vi "quiz1.vi"() -> ()   [LabVIEW 2020]
uses:
  <vilib>/Utility/error.llb/whitespace.ctl
panel:
  in  "Array 3":string[](array[string])
  in  "Array 2":string[](array[string])
  in  "Array":string[](array[string])
  in  "Numeric 2":i64
  out "led 3":bool
  in  "swiche 3":bool
  out "led 2":bool
  in  "swiche 2":bool
  in  "swiche 1":bool
  out "led1":bool
  out "Numeric":i64
  out "number":dbl
  out "Salida de comandos":string
  in  "Ingreso de trama":string
  in  "Ingreso de comandos":string
  in  "Button":bool
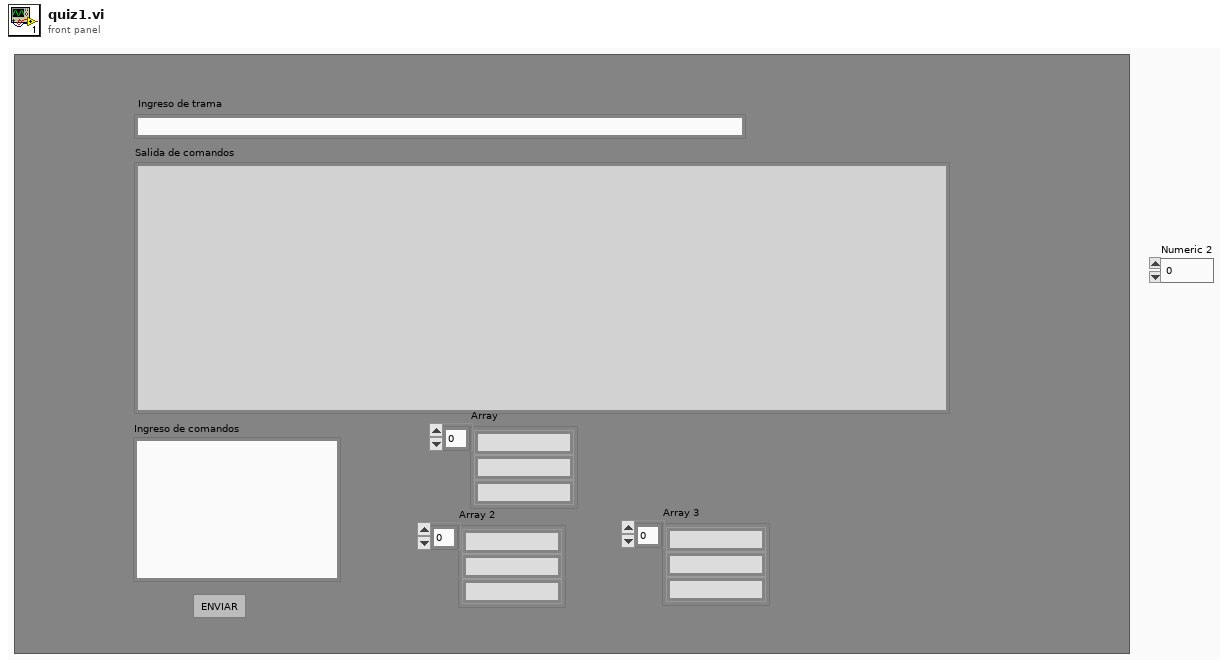
[diagram p1: front panel]
types:
  T1 = enum8{"Enabled", "Disabled", "Disabled and Grayed Out"}
  T2 = typedef "whitespace.ctl" = u16
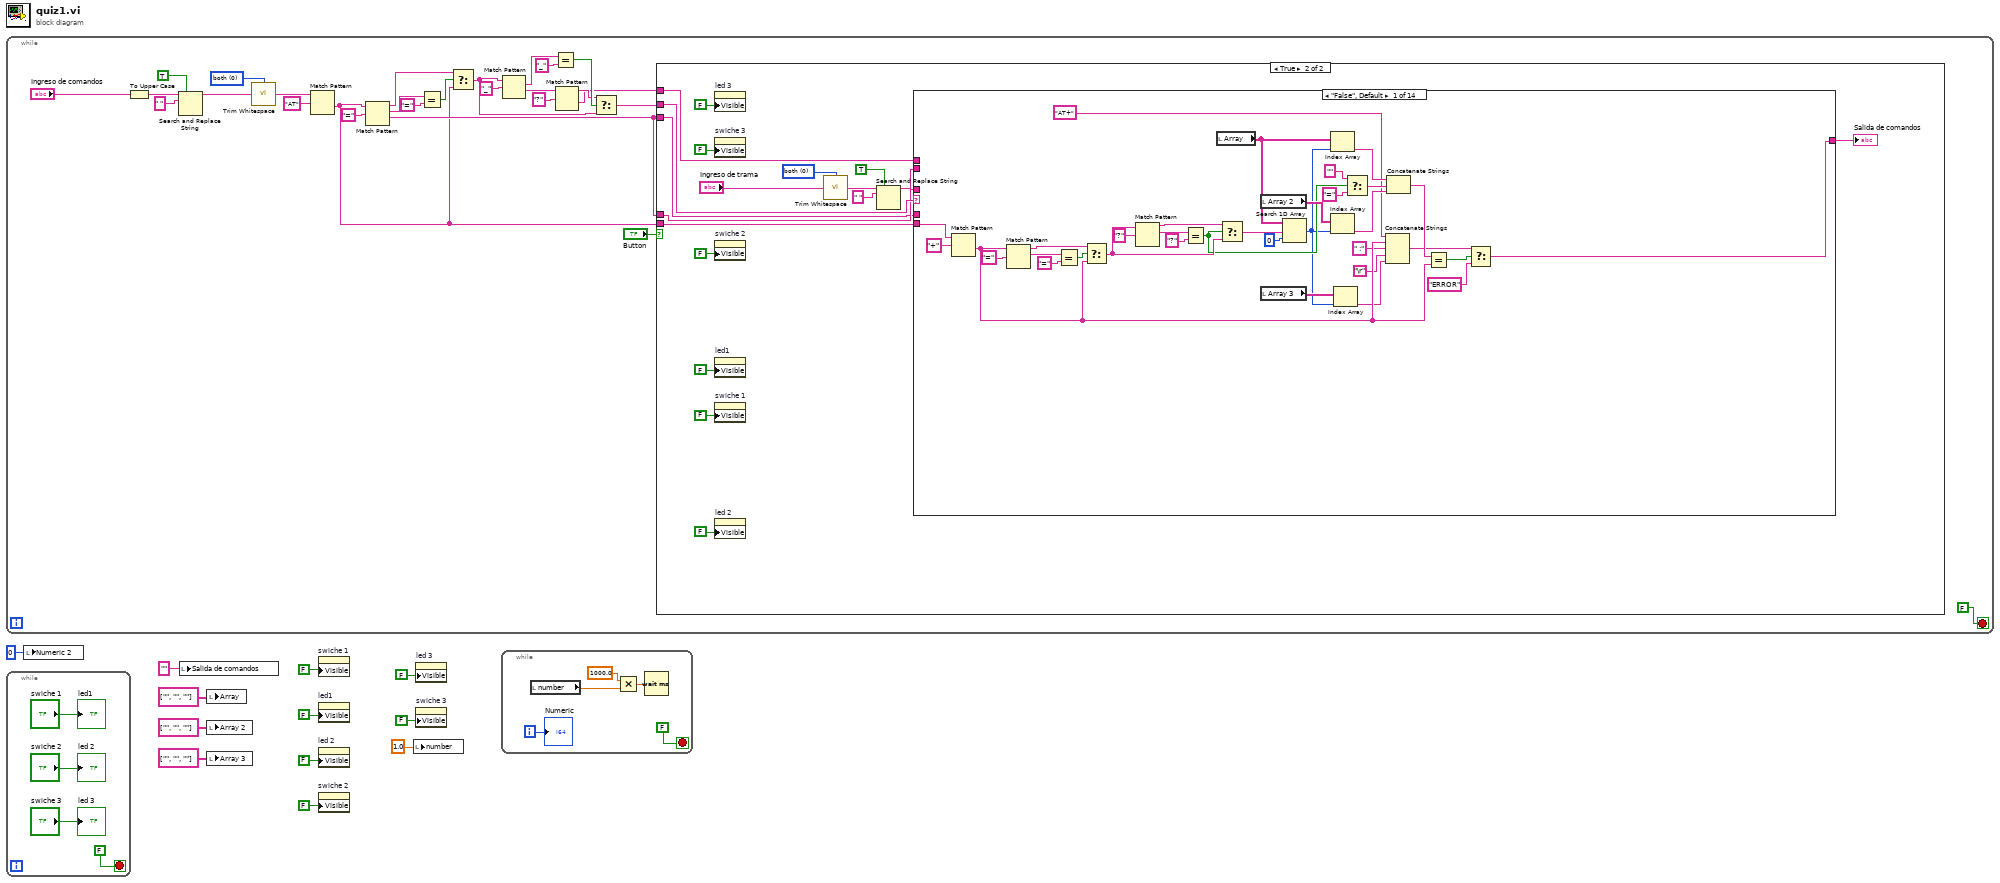
[diagram p0: block diagram]
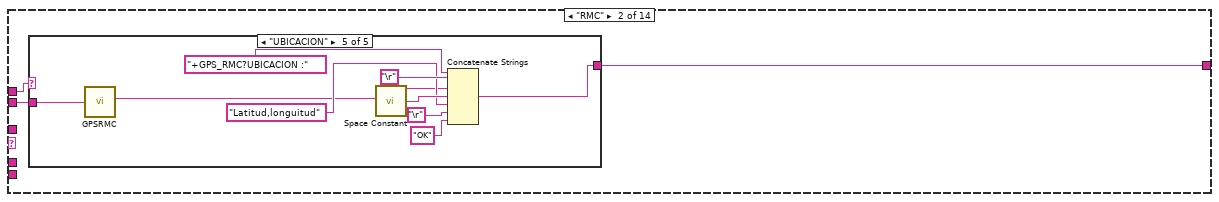
[diagram p3: hidden frame]
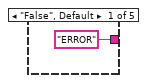
[diagram p4: hidden frame]
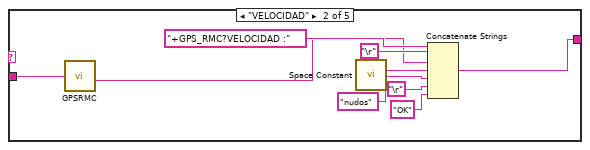
[diagram p5: hidden frame]
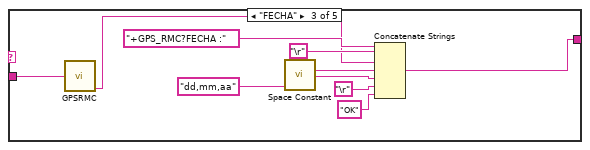
[diagram p6: hidden frame]
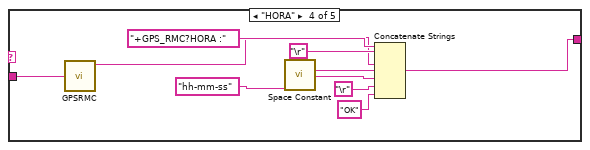
[diagram p7: hidden frame]
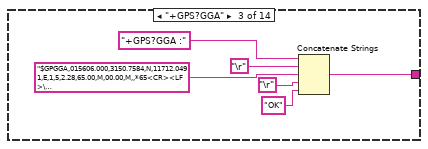
[diagram p8: hidden frame]
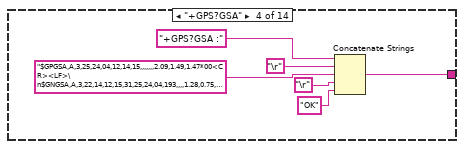
[diagram p9: hidden frame]
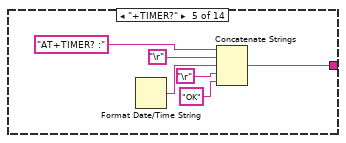
[diagram p10: hidden frame]
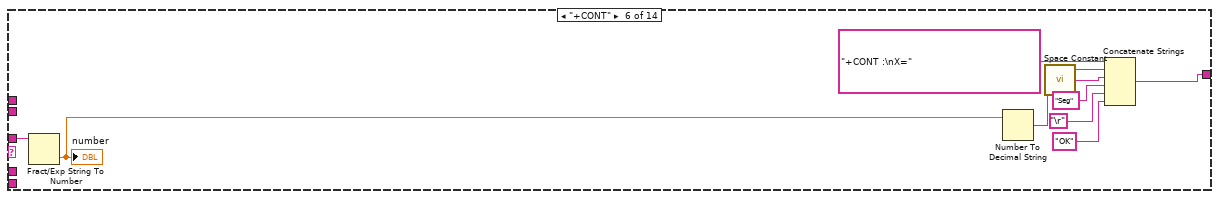
[diagram p11: hidden frame]
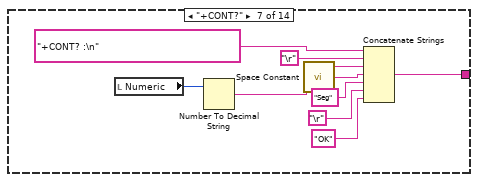
[diagram p12: hidden frame]
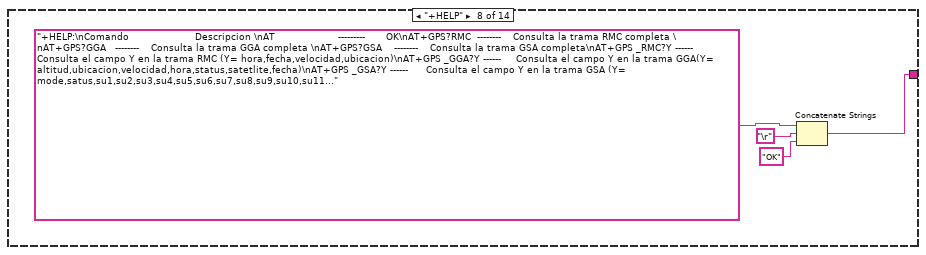
[diagram p13: hidden frame]
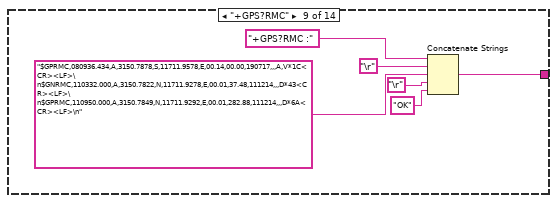
[diagram p14: hidden frame]
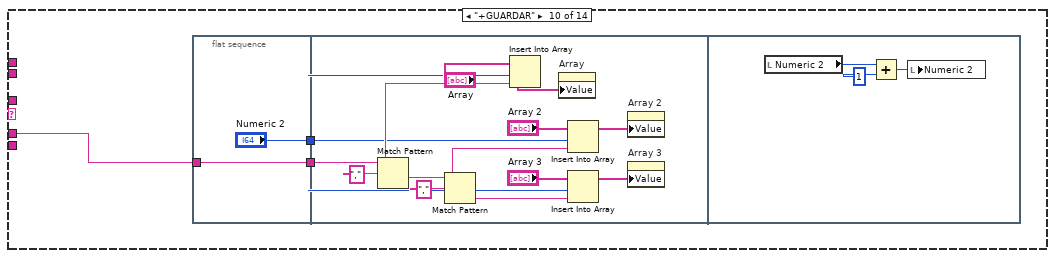
[diagram p15: hidden frame]
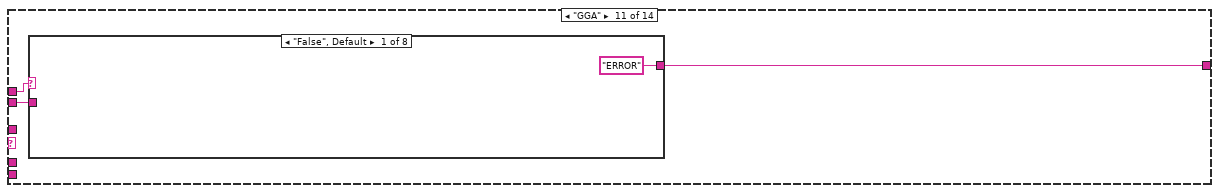
[diagram p16: hidden frame]
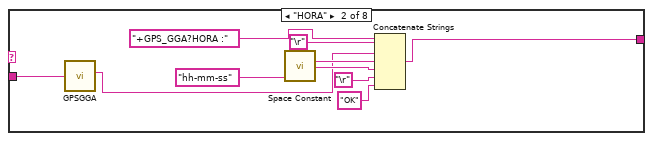
[diagram p17: hidden frame]
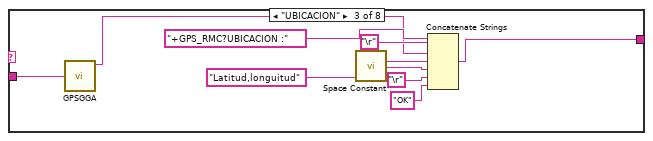
[diagram p18: hidden frame]
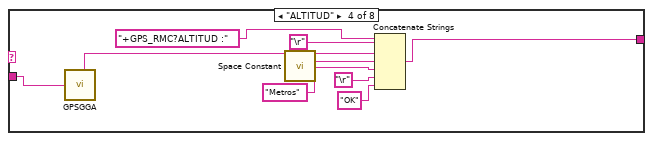
[diagram p19: hidden frame]
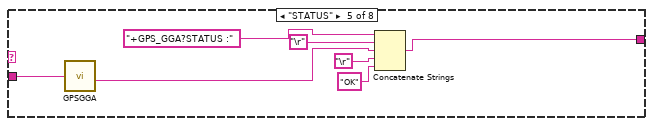
[diagram p20: hidden frame]
diagram:
  n1 = while {
    stop <- FALSE stop-if-true
    w19 = T2 0 items=["both", "start of string", "end of string"] ("location (both)")
    n2 = To Upper Case(1:"Ingreso de comandos") -> (0:w23:string)
    n3 = Search and Replace String(replace all?=TRUE ("replace all? (F)"), input string=w23, search string=" ") -> (result string=w21:string)  [unwired: 5 in, 3 out]
    n4 = call <vilib>:"Trim Whitespace.vi"("string"=w21, "location (both)"=w19) -> ("trimmed string"=w17:string)
    n5 = Match Pattern(string=w17, regular expression="AT") -> (after substring=w13:string)  [unwired: 1 in, 3 out]
    n6 = Match Pattern(string=w13, regular expression="=") -> (before substring=w33:string, match substring=w35:string, after substring=w14:string)  [unwired: 1 in, 1 out]
    n7 = Equal?(x=w35, y="=") -> (x = y?=w32:bool)
    n8 = Select(t=w33, s=w32, f=w13) -> (s? t:f=w27:string)
    n9 = Match Pattern(string=w27, regular expression="_") -> (match substring=w30:string, after substring=w26:string)  [unwired: 1 in, 2 out]
    n10 = Equal?(x=w30, y="_") -> (x = y?=w28:bool)
    n11 = Match Pattern(string=w26, regular expression="?") -> (before substring=w24:string, after substring=w16:string)  [unwired: 1 in, 2 out]
    n12 = Select(t=w24, s=w28, f=w27) -> (s? t:f=w15:string)
    n13 = case shown="True" "Button" {
      tunnel: w14 -> [_ w55]
      tunnel: w15 -> [_ w56]
      tunnel: w16 -> [_ w54]
      tunnel: w14 -> [_ w41]
      tunnel: w13 -> [_ w40]
      frame False {
      }
      frame True {
        w48 = T2 0 items=["both", "start of string", "end of string"] ("location (both)")
        n14 = property on="led 3" class="Bool (strict)"("Visible"=FALSE) -> ()  [unwired: 2 in, 2 out]
        n15 = property on="swiche 3" class="Bool (strict)"("Visible"=FALSE) -> ()  [unwired: 2 in, 2 out]
        n16 = property on="swiche 2" class="Bool (strict)"("Visible"=FALSE) -> ()  [unwired: 2 in, 2 out]
        n17 = property on="led1" class="Bool (strict)"("Visible"=FALSE) -> ()  [unwired: 2 in, 2 out]
        n18 = property on="swiche 1" class="Bool (strict)"("Visible"=FALSE) -> ()  [unwired: 2 in, 2 out]
        n19 = property on="led 2" class="Bool (strict)"("Visible"=FALSE) -> ()  [unwired: 2 in, 2 out]
        n20 = call <vilib>:"Trim Whitespace.vi"("string"="Ingreso de trama", "location (both)"=w48) -> ("trimmed string"=w50:string)
        n21 = Search and Replace String(replace all?=TRUE ("replace all? (F)"), input string=w50, search string=" ") -> (result string=w49:string)  [unwired: 5 in, 3 out]
        n22 = case shown="\"False\", Default" w56 {
          tunnel: [w63 w92 w132 w138 w149 w154 w163 w168 w172 _ w201 w262 w390 w403] -> w57
          tunnel: w49 -> [_ w93 _ _ _ _ _ _ _ _ w200 w260 _ _]
          tunnel: w55 -> [_ _ _ _ _ w158 _ _ _ _ _ _ _ _]
          tunnel: w54 -> [_ w94 _ _ _ _ _ _ _ _ w202 w261 _ _]
          tunnel: w41 -> [_ _ _ _ _ _ _ _ _ w179 _ _ _ _]
          tunnel: w40 -> [w91 _ _ _ _ _ _ _ _ _ _ _ _ _]
          frame "False", Default {
            n23 = Match Pattern(string=w91, regular expression="+") -> (after substring=w65:string)  [unwired: 1 in, 3 out]
            n24 = Match Pattern(string=w65, regular expression="=") -> (before substring=w85:string, match substring=w88:string)  [unwired: 1 in, 2 out]
            n25 = Equal?(x=w88, y="=") -> (x = y?=w86:bool)
            n26 = Select(t=w85, s=w86, f=w65) -> (s? t:f=w78:string)
            n27 = Match Pattern(string=w78, regular expression="?") -> (before substring=w81:string, match substring=w83:string)  [unwired: 1 in, 2 out]
            n28 = Equal?(x=w83, y="?") -> (x = y?=w74:bool)
            n29 = local read "Array"() -> (w77:string[])
            n30 = Select(t=w81, s=w74, f=w78) -> (s? t:f=w80:string)
            n31 = local read "Array 2"() -> (w76:string[])
            n32 = local read "Array 3"() -> (w69:string[])
            n33 = Search 1D Array(1D array=w77, element=w80, start index (0)=0) -> (index of element=w58:i32)
            n34 = Index Array(array=w77, index=w58) -> (element=w75:string)
            n35 = Index Array(array=w76, index=w58) -> (element=w70:string)
            n36 = Index Array(array=w69, index=w58) -> (element=w62:string)
            n37 = Select(t="", s=w74, f="=") -> (s? t:f=w71:string)
            n38 = Concatenate Strings("AT+" ("string"), w65, " :" ("string"), "\r", w62) -> (w64:string)
            n39 = Concatenate Strings(w75, w71, w70) -> (w68:string)
            n40 = Equal?(x=w68, y=w65) -> (x = y?=w67:bool)
            n41 = Select(t=w64, s=w67, f="ERROR") -> (s? t:f=w63:string)
          }
          frame "RMC" {
            n42 = case shown="\"UBICACION\"" w94 {
              tunnel: w93 -> [_ w104 w113 w122 w131]
              tunnel: ["ERROR" w96 w109 w114 w124] -> w92
              frame "False", Default {
              }
              frame "VELOCIDAD" {
                n43 = call "GPSRMC.vi"("String"=w104) -> ("Velocidad"=w100:string)  [unwired: 3 out]
                n44 = call <vilib>:"Space Constant.vi"() -> ("String"=w103:string)
                n45 = Concatenate Strings("+GPS_RMC?VELOCIDAD :", "\r", w100, w103, "nudos" ("string"), "\r", "OK" ("string")) -> (w96:string)
              }
              frame "FECHA" {
                n46 = call "GPSRMC.vi"("String"=w113) -> ("Fecha"=w110:string)  [unwired: 3 out]
                n47 = call <vilib>:"Space Constant.vi"() -> ("String"=w108:string)
                n48 = Concatenate Strings("+GPS_RMC?FECHA :", "\r", w110, w108, "dd,mm,aa" ("string"), "\r", "OK" ("string")) -> (w109:string)
              }
              frame "HORA" {
                n49 = call "GPSRMC.vi"("String"=w122) -> ("Hora"=w115:string)  [unwired: 3 out]
                n50 = call <vilib>:"Space Constant.vi"() -> ("String"=w121:string)
                n51 = Concatenate Strings("+GPS_RMC?HORA :", "\r", w115, w121, "hh-mm-ss" ("string"), "\r", "OK" ("string")) -> (w114:string)
              }
              frame "UBICACION" {
                n52 = call "GPSRMC.vi"("String"=w131) -> ("Ubicación"=w123:string)  [unwired: 3 out]
                n53 = call <vilib>:"Space Constant.vi"() -> ("String"=w130:string)
                n54 = Concatenate Strings("+GPS_RMC?UBICACION :", "\r", w123, w130, "Latitud,longuitud" ("string"), "\r", "OK" ("string")) -> (w124:string)
              }
            }
          }
          frame "+GPS?GGA" {
            n55 = Concatenate Strings("+GPS?GGA :" ("string"), "\r", "$GPGGA,015606.000,3150.7584,N,11712.0491,E,1,5,2.28,65.00,M,00.00,M,,*65<CR><LF>\n$GNGGA,083354.000,3150.7790,N,11711.9289,E,1,8,2.85,53.20,M,00.00,M,,*4B<CR><LF>", "\r", "OK" ("string")) -> (w132:string)
          }
          frame "+GPS?GSA" {
            n56 = Concatenate Strings("+GPS?GSA :" ("string"), "\r", "$GPGSA,A,3,25,24,04,12,14,15,,,,,,,2.09,1.49,1.47*00<CR><LF>\n$GNGSA,A,3,22,14,12,15,31,25,24,04,193,,,,1.28,0.75,1.03*29<CR><LF>\n$GPGSA,A,3,03,17,09,23,,,,,,,,,3.65,3.51,0.99,1*15<CR><LF>\n$GNGSA,A,3,09,17,19,06,23,,,,,,,,2.20,1.97,0.98,1*0F<CR><LF>", "\r", "OK" ("string")) -> (w138:string)
          }
          frame "+TIMER?" {
            n57 = Format Date/Time String() -> (date/time string=w146:string)  [unwired: 3 in]
            n58 = Concatenate Strings("AT+TIMER? :", "\r", w146, "\r", "OK" ("string")) -> (w149:string)
          }
          frame "+CONT" {
            n59 = Fract/Exp String To Number(string=w158) -> (number=w156:dbl)  [unwired: 3 in, 1 out]
            "number" <- w156
            n60 = Number To Decimal String(number=w156) -> (decimal integer string=w155:string)  [unwired: 1 in]
            n61 = call <vilib>:"Space Constant.vi"() -> ("String"=w153:string)
            n62 = Concatenate Strings("+CONT :\nX=", w155, w153, "Seg" ("string"), "\r", "OK" ("string")) -> (w154:string)
          }
          frame "+CONT?" {
            n63 = local read "Numeric"() -> (w167:i64)
            n64 = Number To Decimal String(number=w167) -> (decimal integer string=w164:string)  [unwired: 1 in]
            n65 = call <vilib>:"Space Constant.vi"() -> ("String"=w159:string)
            n66 = Concatenate Strings("+CONT? :\n", "\r", w164, w159, "Seg" ("string"), "\r", "OK" ("string")) -> (w163:string)
          }
          frame "+HELP" {
            n67 = Concatenate Strings("+HELP:\nComando                      Descripcion \nAT                     ---------       OK\nAT+GPS?RMC  --------    Consulta la trama RMC completa \nAT+GPS?GGA   --------    Consulta la trama GGA completa \nAT+GPS?GSA    --------    Consulta la trama GSA completa\nAT+GPS _RMC?Y ------    Consulta el campo Y en la trama RMC (Y= hora,fecha,velocidad,ubicacion)\nAT+GPS _GGA?Y ------     Consulta el campo Y en la trama GGA(Y= altitud,ubicacion,velocidad,hora,status,satetlite,fecha)\nAT+GPS _GSA?Y ------      Consulta el campo Y en la trama GSA (Y= mode,satus,su1,su2,su3,su4,su5,su6,su7,su8,su9,su10,su11,su12)\nAT+TIMER?           --------  Consulta la hora y fecha del sistema\nAT+CONT=X      --------- Modifica el tiempo de incremento del contador en X tiempo \nAT+CONT?         ----------Lee  la variable del contador \nAT+ESTADO?     ----------Lee el estado de los leds y pulsadores\nAT+CAMBIAR   ---------  Modifica el estado de los leds y el pulsador", "\r", "OK" ("string")) -> (w168:string)
          }
          frame "+GPS?RMC" {
            n68 = Concatenate Strings("+GPS?RMC :" ("string"), "\r", "$GPRMC,080936.434,A,3150.7878,S,11711.9578,E,00.14,00.00,190717,,,A,V*1C<CR><LF>\n$GNRMC,110332.000,A,3150.7822,N,11711.9278,E,00.01,37.48,111214,,,D*43<CR><LF>\n$GPRMC,110950.000,A,3150.7849,N,11711.9292,E,00.01,282.88,111214,,,D*6A<CR><LF>\n", "\r", "OK" ("string")) -> (w172:string)
          }
          frame "+GUARDAR" {
            n69 = flat-sequence {
              tunnel: ["Numeric 2"] -> w180
              tunnel: w179 -> [w181]
              tunnel: [w181] -> w178
              tunnel: w180 -> [w184]
              tunnel: w178 -> [w196]
              frame #0 {
              }
              frame #1 {
                n70 = Match Pattern(string=w196, regular expression=",") -> (before substring=w194:string, after substring=w189:string)  [unwired: 1 in, 2 out]
                n71 = Match Pattern(string=w189, regular expression=",") -> (before substring=w187:string, after substring=w185:string)  [unwired: 1 in, 2 out]
                n72 = Insert Into Array(array="Array", index=w184, new element=w194) -> (w191:string[])
                n73 = property on="Array" class="Arr (strict)"("Value"=w191) -> ()  [unwired: 2 in, 2 out]
                n74 = Insert Into Array(array="Array 2", index=w184, new element=w187) -> (w190:string[])
                n75 = Insert Into Array(array="Array 3", index=w184, new element=w185) -> (w183:string[])
                n76 = property on="Array 2" class="Arr (strict)"("Value"=w190) -> ()  [unwired: 2 in, 2 out]
                n77 = property on="Array 3" class="Arr (strict)"("Value"=w183) -> ()  [unwired: 2 in, 2 out]
              }
              frame #2 {
                n78 = local read "Numeric 2"() -> (w199:i64)
                n79 = Add(x=w199, y=i64 1) -> (x+y=w197:i64)
                n80 = local write "Numeric 2"(w197) -> ()
              }
            }
          }
          frame "GGA" {
            n81 = case shown="\"False\", Default" w202 {
              tunnel: ["ERROR" w206 w214 w222 w233 w238 w248 w254] -> w201
              tunnel: w200 -> [_ w204 w213 w223 w237 w246 w253 _]
              frame "False", Default {
              }
              frame "HORA" {
                n82 = call "GPSGGA.vi"("String"=w204) -> ("Hora"=w205:string)  [unwired: 5 out]
                n83 = call <vilib>:"Space Constant.vi"() -> ("String"=w212:string)
                n84 = Concatenate Strings("+GPS_GGA?HORA :", "\r", w205, w212, "hh-mm-ss" ("string"), "\r", "OK" ("string")) -> (w206:string)
              }
              frame "UBICACION" {
                n85 = call "GPSGGA.vi"("String"=w213) -> ("Ubicación"=w215:string)  [unwired: 5 out]
                n86 = call <vilib>:"Space Constant.vi"() -> ("String"=w221:string)
                n87 = Concatenate Strings("+GPS_RMC?UBICACION :", "\r", w215, w221, "Latitud,longuitud" ("string"), "\r", "OK" ("string")) -> (w214:string)
              }
              frame "ALTITUD" {
                n88 = call "GPSGGA.vi"("String"=w223) -> ("Altitud"=w224:string)  [unwired: 5 out]
                n89 = call <vilib>:"Space Constant.vi"() -> ("String"=w230:string)
                n90 = Concatenate Strings("+GPS_RMC?ALTITUD :", "\r", w224, w230, "Metros" ("string"), "\r", "OK" ("string")) -> (w222:string)
              }
              frame "STATUS" {
                n91 = call "GPSGGA.vi"("String"=w237) -> ("Fix Status"=w236:string)  [unwired: 5 out]
                n92 = Concatenate Strings("+GPS_GGA?STATUS :" ("string"), "\r", w236, "\r", "OK" ("string")) -> (w233:string)
              }
              frame "GEOIDE" {
                n93 = call "GPSGGA.vi"("String"=w246) -> ("Sep Geoide"=w239:string)  [unwired: 5 out]
                n94 = call <vilib>:"Space Constant.vi"() -> ("String"=w245:string)
                n95 = Concatenate Strings("+GPS_RMC?GEOIDE :", "\r", w239, w245, "Metros" ("string"), "\r", "OK" ("string")) -> (w238:string)
              }
              frame "SATELITE" {
                n96 = call "GPSGGA.vi"("String"=w253) -> ("# Satelite"=w249:string)  [unwired: 5 out]
                n97 = Concatenate Strings("+GPS_GGA?SATELITE :" ("string"), "\r", w249, "\r", "OK" ("string")) -> (w248:string)
              }
              frame "VELOCIDAD" {
                n98 = Concatenate Strings("+GPS_GGA?VELOCIDAD :" ("string"), "\r", "La trama GGA no tiene velocidad", "\r", "OK" ("string")) -> (w254:string)
              }
            }
          }
          frame "GSA" {
            n99 = case shown="\"False\", Default" w261 {
              tunnel: ["ERROR -CAMPO NO ENCONTRADO" w265 w274 w282 w291 w300 w310 w319 w328 w336 w345 w355 w363 w372 w382] -> w262
              tunnel: w260 -> [_ w264 w273 w283 w292 w301 w309 w318 w327 w337 w346 w354 w364 w373 w381]
              frame "False", Default {
              }
              frame "MODO" {
                n100 = call "GPSGSA.vi"("string"=w264) -> ("Array"=w272:string[])
                n101 = Index Array(array=w272, index=0) -> (element=w266:string)
                n102 = Concatenate Strings("+GPS_GSA?MODO :" ("string"), "\r", w266, "\r", "OK" ("string")) -> (w265:string)
              }
              frame "STATUS" {
                n103 = call "GPSGSA.vi"("string"=w273) -> ("Array"=w281:string[])
                n104 = Index Array(array=w281, index=1) -> (element=w275:string)
                n105 = Concatenate Strings("+GPS_GSA?STATUS :" ("string"), "\r", w275, "\r", "OK" ("string")) -> (w274:string)
              }
              frame "SATELITE1" {
                n106 = call "GPSGSA.vi"("string"=w283) -> ("Array"=w290:string[])
                n107 = Index Array(array=w290, index=2) -> (element=w284:string)
                n108 = Concatenate Strings("+GPS_GSA?SATELITE1 :" ("string"), "\r", w284, "\r", "OK" ("string")) -> (w282:string)
              }
              frame "SATELITE2" {
                n109 = call "GPSGSA.vi"("string"=w292) -> ("Array"=w299:string[])
                n110 = Index Array(array=w299, index=3) -> (element=w293:string)
                n111 = Concatenate Strings("+GPS_GSA?SATELITE2 :" ("string"), "\r", w293, "\r", "OK" ("string")) -> (w291:string)
              }
              frame "SATELITE3" {
                n112 = call "GPSGSA.vi"("string"=w301) -> ("Array"=w308:string[])
                n113 = Index Array(array=w308, index=4) -> (element=w302:string)
                n114 = Concatenate Strings("+GPS_GSA?SATELITE3 :" ("string"), "\r", w302, "\r", "OK" ("string")) -> (w300:string)
              }
              frame "SATELITE4" {
                n115 = call "GPSGSA.vi"("string"=w309) -> ("Array"=w317:string[])
                n116 = Index Array(array=w317, index=5) -> (element=w311:string)
                n117 = Concatenate Strings("+GPS_GSA?SATELITE4 :" ("string"), "\r", w311, "\r", "OK" ("string")) -> (w310:string)
              }
              frame "SATELITE5" {
                n118 = call "GPSGSA.vi"("string"=w318) -> ("Array"=w326:string[])
                n119 = Index Array(array=w326, index=6) -> (element=w320:string)
                n120 = Concatenate Strings("+GPS_GSA?SATELITE5 :" ("string"), "\r", w320, "\r", "OK" ("string")) -> (w319:string)
              }
              frame "SATELITE9" {
                n121 = call "GPSGSA.vi"("string"=w327) -> ("Array"=w335:string[])
                n122 = Index Array(array=w335, index=10) -> (element=w329:string)
                n123 = Concatenate Strings("+GPS_GSA?SATELITE9 :" ("string"), "\r", w329, "\r", "OK" ("string")) -> (w328:string)
              }
              frame "SATELITE11" {
                n124 = call "GPSGSA.vi"("string"=w337) -> ("Array"=w344:string[])
                n125 = Index Array(array=w344, index=12) -> (element=w338:string)
                n126 = Concatenate Strings("+GPS_GSA?SATELITE11 :" ("string"), "\r", w338, "\r", "OK" ("string")) -> (w336:string)
              }
              frame "SATELITE10" {
                n127 = call "GPSGSA.vi"("string"=w346) -> ("Array"=w353:string[])
                n128 = Index Array(array=w353, index=11) -> (element=w347:string)
                n129 = Concatenate Strings("+GPS_GSA?SATELITE10 :" ("string"), "\r", w347, "\r", "OK" ("string")) -> (w345:string)
              }
              frame "SATELITE12" {
                n130 = call "GPSGSA.vi"("string"=w354) -> ("Array"=w362:string[])
                n131 = Index Array(array=w362, index=13) -> (element=w356:string)
                n132 = Concatenate Strings("+GPS_GSA?SATELITE12 :" ("string"), "\r", w356, "\r", "OK" ("string")) -> (w355:string)
              }
              frame "SATELITE7" {
                n133 = call "GPSGSA.vi"("string"=w364) -> ("Array"=w371:string[])
                n134 = Index Array(array=w371, index=8) -> (element=w365:string)
                n135 = Concatenate Strings("+GPS_GSA?SATELITE7 :" ("string"), "\r", w365, "\r", "OK" ("string")) -> (w363:string)
              }
              frame "SATELITE6" {
                n136 = call "GPSGSA.vi"("string"=w373) -> ("Array"=w380:string[])
                n137 = Index Array(array=w380, index=7) -> (element=w374:string)
                n138 = Concatenate Strings("+GPS_GSA?SATELITE6 :" ("string"), "\r", w374, "\r", "OK" ("string")) -> (w372:string)
              }
              frame "SATELITE8" {
                n139 = call "GPSGSA.vi"("string"=w381) -> ("Array"=w389:string[])
                n140 = Index Array(array=w389, index=9) -> (element=w383:string)
                n141 = Concatenate Strings("+GPS_GSA?SATELITE8 :" ("string"), "\r", w383, "\r", "OK" ("string")) -> (w382:string)
              }
            }
          }
          frame "+ESTADO?" {
            n142 = property on="swiche 1" class="Bool (strict)"("Visible"=TRUE) -> ()  [unwired: 2 in, 2 out]
            n143 = property on="swiche 2" class="Bool (strict)"("Visible"=TRUE) -> ()  [unwired: 2 in, 2 out]
            n144 = property on="swiche 3" class="Bool (strict)"("Visible"=TRUE) -> ()  [unwired: 2 in, 2 out]
            n145 = property on="led 3" class="Bool (strict)"("Visible"=TRUE) -> ()  [unwired: 2 in, 2 out]
            n146 = property on="led 2" class="Bool (strict)"("Visible"=TRUE) -> ()  [unwired: 2 in, 2 out]
            n147 = property on="led1" class="Bool (strict)"("Visible"=TRUE) -> ()  [unwired: 2 in, 2 out]
            n148 = property on="swiche 3" class="Bool (strict)"("DisabledEnum"=T1."Disabled" ("Disabled")) -> ()  [unwired: 2 in, 2 out]
            n149 = property on="swiche 2" class="Bool (strict)"("DisabledEnum"=T1."Disabled" ("Disabled")) -> ()  [unwired: 2 in, 2 out]
            n150 = property on="swiche 1" class="Bool (strict)"("DisabledEnum"=T1."Disabled" ("Disabled")) -> ()  [unwired: 2 in, 2 out]
            n151 = Concatenate Strings("AT+ESTADO? :", "\r", "OK" ("string")) -> (w390:string)
          }
          frame "+CAMBIAR" {
            n152 = property on="swiche 3" class="Bool (strict)"("Visible"=TRUE) -> ()  [unwired: 2 in, 2 out]
            n153 = property on="led 3" class="Bool (strict)"("Visible"=TRUE) -> ()  [unwired: 2 in, 2 out]
            n154 = property on="swiche 2" class="Bool (strict)"("Visible"=TRUE) -> ()  [unwired: 2 in, 2 out]
            n155 = property on="led1" class="Bool (strict)"("Visible"=TRUE) -> ()  [unwired: 2 in, 2 out]
            n156 = property on="swiche 1" class="Bool (strict)"("Visible"=TRUE) -> ()  [unwired: 2 in, 2 out]
            n157 = property on="led 2" class="Bool (strict)"("Visible"=TRUE) -> ()  [unwired: 2 in, 2 out]
            n158 = property on="swiche 3" class="Bool (strict)"("DisabledEnum"=T1."Enabled" ("Disabled")) -> ()  [unwired: 2 in, 2 out]
            n159 = property on="swiche 2" class="Bool (strict)"("DisabledEnum"=T1."Enabled" ("Disabled")) -> ()  [unwired: 2 in, 2 out]
            n160 = property on="swiche 1" class="Bool (strict)"("DisabledEnum"=T1."Enabled" ("Disabled")) -> ()  [unwired: 2 in, 2 out]
            n161 = Concatenate Strings("AT+CAMBIAR :", "\r", "OK" ("string")) -> (w403:string)
          }
        }
        "Salida de comandos" <- w57
      }
    }
  }
  n162 = while {
    stop <- FALSE stop-if-true
    "led1" <- "swiche 1"
    "led 2" <- "swiche 2"
    "led 3" <- "swiche 3"
  }
  n163 = local write "Numeric 2"(i64 0 ("Numeric 2")) -> ()
  n164 = local write "Salida de comandos"("" ("String 2")) -> ()
  n165 = local write "Array"(string[] ["", "", ""] ("Array")) -> ()
  n166 = local write "Array 2"(string[] ["", "", ""] ("Array 2")) -> ()
  n167 = local write "Array 3"(string[] ["", "", ""] ("Array 3")) -> ()
  n168 = property on="swiche 1" class="Bool (strict)"("Visible"=FALSE) -> ()  [unwired: 2 in, 2 out]
  n169 = property on="led1" class="Bool (strict)"("Visible"=FALSE) -> ()  [unwired: 2 in, 2 out]
  n170 = property on="led 2" class="Bool (strict)"("Visible"=FALSE) -> ()  [unwired: 2 in, 2 out]
  n171 = property on="swiche 2" class="Bool (strict)"("Visible"=FALSE) -> ()  [unwired: 2 in, 2 out]
  n172 = local write "number"(1.0 ("number")) -> ()
  n173 = property on="led 3" class="Bool (strict)"("Visible"=FALSE) -> ()  [unwired: 2 in, 2 out]
  n174 = property on="swiche 3" class="Bool (strict)"("Visible"=FALSE) -> ()  [unwired: 2 in, 2 out]
  n175 = while {
    i -> [w421]
    stop <- FALSE stop-if-true
    n176 = local read "number"() -> (w422:dbl)
    n177 = Multiply(x=1000.0, y=w422) -> (x*y=w424:dbl)
    n178 = Wait (ms)(milliseconds to wait=w424) -> ()  [unwired: 1 out]
    "Numeric" <- w421
  }
